vi "advanced_cont_memtest_1channel-v05justNoise.vi"(0 "Pulse AI task in":refnum<k21>, 1 "replicates":i32=5, 4 "Pulse AO task in":refnum<k21>, 5 "error in":errorcluster, 7 "memtest":T2={"Samples to Read"=1000, "Rate (Hz)"=20000.0, "Amplitude (mV/pA)"=10.0, "Offset (mV/pA)"=-60.0, "Frequency (Hz)"=-60.0, "duty cycle (%)"=50.0, "phase"=0.0} {"phase" format="%.2p"; "duty cycle (%)" format="%0.2f"}, 11 "which clamp":enum16{"VClamp", "IClamp"}(ring)) -> (9 "Power Spectrum":dbl[](graph), 13 "avg peak height":dbl, 14 "Pulse AI task out":refnum<k21>, 15 "data out (pA or mV)":waveform(dbl)[](graph), 16 "cell stats":T1 {"STD" format="%010.2f"; "Variance" format="%010.2f"; "Rt (MOhms)" format="%010.2f"; "tau (ms)" format="%08.2g"; "Cm (pF)" format="%08.2f"; "Ra (MOhms)" format="%010.2f"; "Rm (MOhms)" format="%010.2f"; "Ihold (pA)" format="%010.2f"}, 17 "cont memtest error?":bool, 18 "Pulse AO task out":refnum<k21>, 19 "error out":errorcluster)   [LabVIEW 2015]
uses:
  <resource>/objmgr/daqmx.rc
  wc_protocol_v1.003 Folder/whole_cell_protocol/Controls/cell_stats-v02.ctl
  <vilib>/DAQmx/read.llb/DAQmx Read (Analog Wfm 1Chan NSamp).vi
  controls/memtest_def.ctl
panel:
  out "AvailSampPerChan":u32
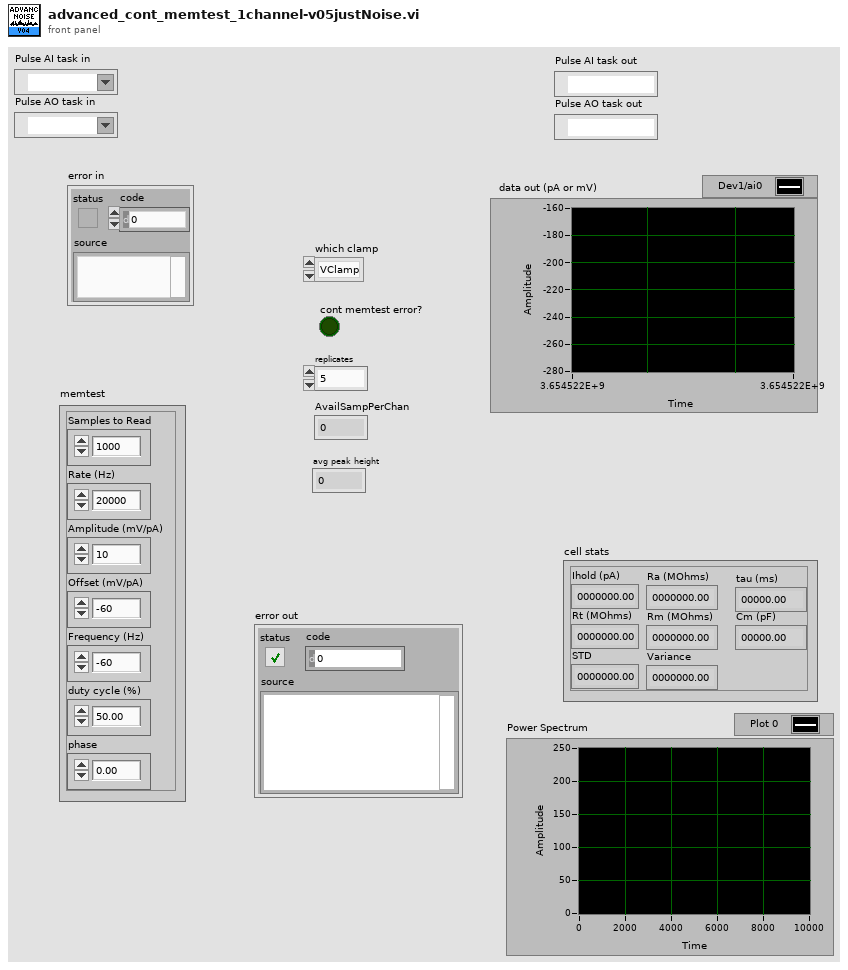
[diagram p1: front panel]
types:
  T1 = typedef "cell_stats-v02.ctl" = cluster{"Ihold (pA)":dbl, "Rm (MOhms)":dbl, "Ra (MOhms)":dbl, "Cm (pF)":dbl, "tau (ms)":dbl, "Rt (MOhms)":dbl, "Variance":dbl, "STD":dbl}
  T2 = typedef "memtest_def.ctl" = cluster{"Samples to Read":i32, "Rate (Hz)":dbl, "Amplitude (mV/pA)":dbl, "Offset (mV/pA)":dbl, "Frequency (Hz)":dbl, "duty cycle (%)":dbl, "phase":dbl}
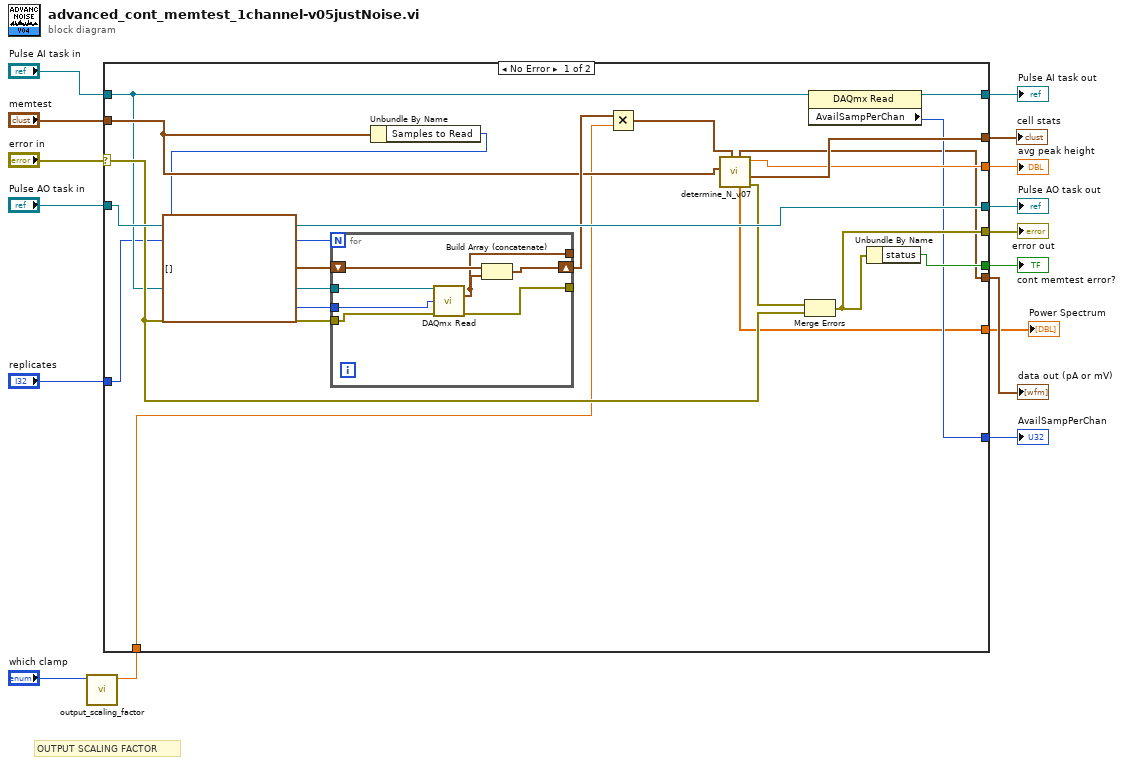
[diagram p0: block diagram]
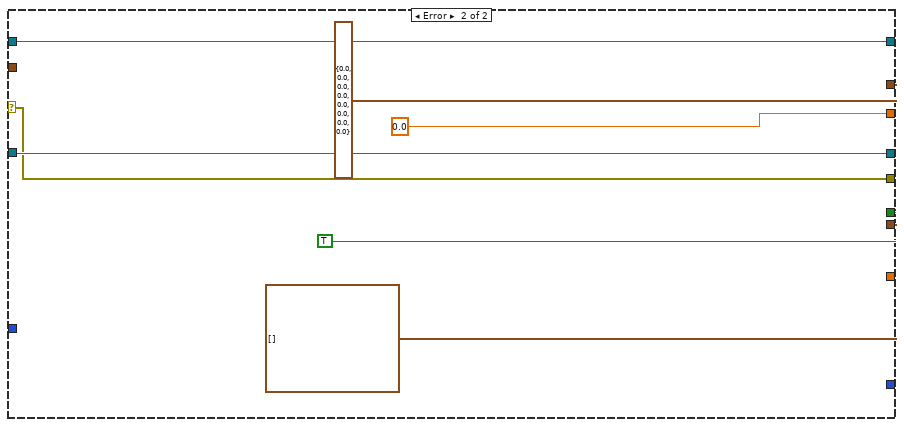
[diagram p2: hidden frame]
diagram:
  # "OUTPUT SCALING FACTOR"
  n1 = call "output_scaling_factor.vi"("which clamp"="which clamp") -> ("output scaling factor"=w9:dbl)  [unwired: 10 in]
  n2 = case shown="No Error" "error in" {
    selector: "error in" -> [w30 w46]
    tunnel: "Pulse AI task in" -> [w25 w48]
    tunnel: "Pulse AO task in" -> [w35 w47]
    tunnel: [w31 TRUE ("status")] -> w13
    tunnel: [w35 w47] -> w12
    tunnel: [w34 w48] -> w11
    tunnel: [w32 w46] -> w10
    tunnel: w9 -> [w23 _]
    tunnel: [w27 0.0 ("avg peak height")] -> w6
    tunnel: [w28 T1 {"Ihold (pA)"=0.0, "Rm (MOhms)"=0.0, "Ra (MOhms)"=0.0, "Cm (pF)"=0.0, "tau (ms)"=0.0, "Rt (MOhms)"=0.0, "Variance"=0.0, "STD"=0.0} ("cell stats")] -> w7
    tunnel: "replicates" -> [w20 _]
    tunnel: "memtest" -> [w26 _]
    tunnel: [w17 waveform(dbl)[] []] -> w3
    tunnel: [w24 _] -> w2
    tunnel: [w19 _] -> w1
    frame No Error {
      n3 = Unbundle By Name(w26) -> ("Samples to Read"=w21:i32)
      n4 = for {
        N: w20 -> [_]
        tunnel: w25 -> [w42]
        tunnel: w21 -> [w41]
        tunnel: w30 -> [w40]
        tunnel: [w37] -> _
        shift-right: [w39] -> w29
        shift-left: waveform(dbl)[] [] -> [w38]
        tunnel: [w36] -> _
        n5 = call-poly <vilib>:"DAQmx Read.vi"("task/channels in"=w42, "number of samples per channel"=w41, "error in"=w40) -> ("data"=w36:waveform(dbl), "error out"=w37:errorcluster)  [unwired: 10 in, 1 out]
        n6 = Build Array (concatenate)(w38, w36) -> (w39:waveform(dbl)[])
      }
      n7 = Multiply(x=w29, y=w23) -> (x*y=w18:waveform(dbl)[])
      n8 = call "determine_N_v07.vi"("memtest"=w26, "Noise Data in (pA)"=w18) -> ("Waveform Graph"=w17:waveform(dbl)[], "Power Spectrum"=w19:dbl[], "avg peak height"=w27:dbl, "cell stats"=w28:T1, "error out"=w33:errorcluster)  [unwired: 3 in, 1 out]
      n9 = Merge Errors(w33, w30) -> (w32:errorcluster)
      n10 = property class="DAQmx Read"(reference=w25) -> (reference out=w34:refnum<k21>, "AvailSampPerChan"=w24:u32)  [unwired: 1 in, 1 out]
      n11 = Unbundle By Name(w32) -> ("status"=w31:bool)
    }
    frame Error {
    }
  }
  "Pulse AI task out" <- w11
  "Pulse AO task out" <- w12
  "cont memtest error?" <- w13
  "error out" <- w10
  "cell stats" <- w7
  "avg peak height" <- w6
  "data out (pA or mV)" <- w3
  "AvailSampPerChan" <- w2
  "Power Spectrum" <- w1
